vi "recordResultsToFile.vi"(8 "error in (no error)":errorcluster, 10 "Results":variant, 11 "ImageAnalyser in":refnum<class "ImageAnalyser.lvclass">) -> (0 "error out":errorcluster, 3 "ImageAnalyser out":refnum<class "ImageAnalyser.lvclass">)   [LabVIEW 2009, in "Tools.lvlib" / "Imaging.lvlib" / "ImageAnalyser.lvclass"]
uses:
  ImageAnalyser.lvclass
  Filing/FileNeologist/FileNeologist.lvclass
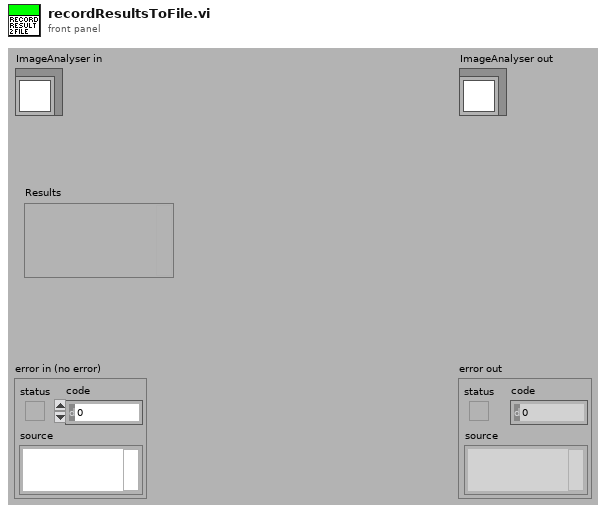
[diagram p1: front panel]
types:
  T1 = cluster{"Name":string, "Results":dbl[], "AnalysisType":string}
  T2 = enum16{"open", "replace", "create", "open or create", "replace or create", "replace or create with confirmation"}
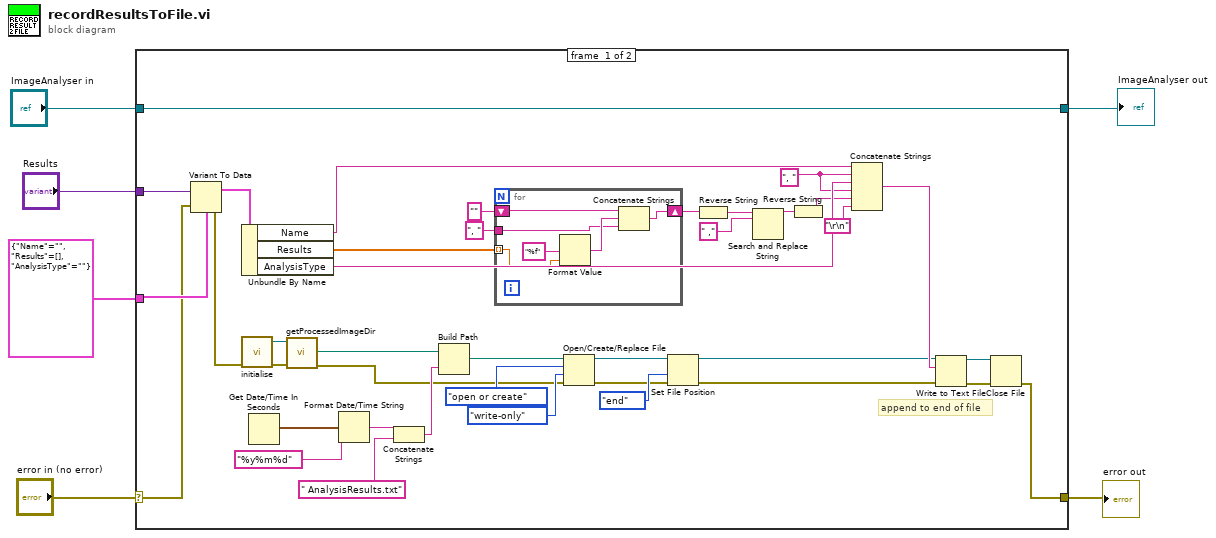
[diagram p0: block diagram]
diagram:
  n1 = case shown="No Error" "error in (no error)" {
    selector: "error in (no error)" -> [w41 w53]
    tunnel: [w11 w53] -> w5
    tunnel: [w45 w52] -> w3
    tunnel: "ImageAnalyser in" -> [w45 w52]
    tunnel: "Results" -> [w44 _]
    tunnel: T1 {"Name"="", "Results"=[], "AnalysisType"=""} ("output cluster") -> [w43 _]
    frame #0 {
      w22 = ", "
      # "append to end of file"
      n2 = Variant To Data(error in=w41, Variant=w44, type=w43) -> (error out=w38:errorcluster, data=w42:T1)
      n3 = Unbundle By Name(w42) -> ("Name"=w25:string, "Results"=w31:dbl[], "AnalysisType"=w23:string)
      n4 = call "initialise.vi"("error in (no error)"=w38) -> ("error out"=w39:errorcluster, "FileNeologist out"=w40:refnum<class "FileNeologist.lvclass">)  [unwired: 9 in]
      n5 = Get Date/Time In Seconds() -> (seconds since 1Jan1904=w36:timestamp)
      n6 = call-dynamic "getProcessedImageDir.vi"("error in (no error)"=w39, "FileNeologist in"=w40) -> ("error out"=w14:errorcluster, "Path"=w37:path)  [unwired: 7 in, 1 out]
      n7 = Format Date/Time String(time format string (%c)="%y%m%d", seconds (now)=w36) -> (date/time string=w34:string)  [unwired: 1 in]
      n8 = Concatenate Strings(w34, " AnalysisResults.txt") -> (w32:string)
      n9 = Build Path(base path=w37, name or relative path=w32) -> (appended path=w18:path)
      n10 = for {
        tunnel: w31 -> [w50] mode=indexing
        shift-right: [w47] -> w29
        shift-left: "" -> [w49]
        tunnel: ", " -> [w46]
        n11 = Format Value(format string="%f", value (0)=w50) -> (output string=w48:string)  [unwired: 1 in]
        n12 = Concatenate Strings(w49, w48, w46) -> (w47:string)
      }
      n13 = Open/Create/Replace File(file path (use dialog)=w18, error in=w14, operation (0:open)=T2."open or create", access (0:read/write)=enum16{"read/write", "read-only", "write-only"}."write-only") -> (refnum out=w17:refnum<file>, error out=w8:errorcluster)  [unwired: 2 in, 1 out]
      n14 = Set File Position(refnum=w17, from (0:start)=enum16{"start", "end", "current"}."end", error in=w8) -> (refnum out=w10:refnum<file>, error out=w7:errorcluster)  [unwired: 1 in]
      n15 = Reverse String(1:w29) -> (0:w28:string)
      n16 = Search and Replace String(input string=w28, search string=" ,") -> (result string=w26:string)  [unwired: 6 in, 3 out]
      n17 = Reverse String(1:w26) -> (0:w21:string)
      n18 = Concatenate Strings(w25, w22, w23, w22, w21, "\r\n") -> (w19:string)
      n19 = Write to Text File(file (use dialog)=w10, text=w19, error in=w7) -> (refnum out=w12:refnum<file>, error out=w13:errorcluster)  [unwired: 1 in, 1 out]
      n20 = Close File(refnum=w12, error in=w13) -> (error out=w11:errorcluster)  [unwired: 1 out]
    }
    frame #1 {
    }
  }
  "error out" <- w5
  "ImageAnalyser out" <- w3
